vi "Graficar.vi"(8 "error in":errorcluster, 10 "group name":string, 11 "channel name":string) -> (0 "error out":errorcluster, 2 "XY Graph":cluster{timestamp[], dbl[]}(graph), 3 "semaphore out":T1)   [LabVIEW 2015]
panel:
  out "x-y":i32
  out "count":i32
  out "Boolean":bool
  out "offset":i32
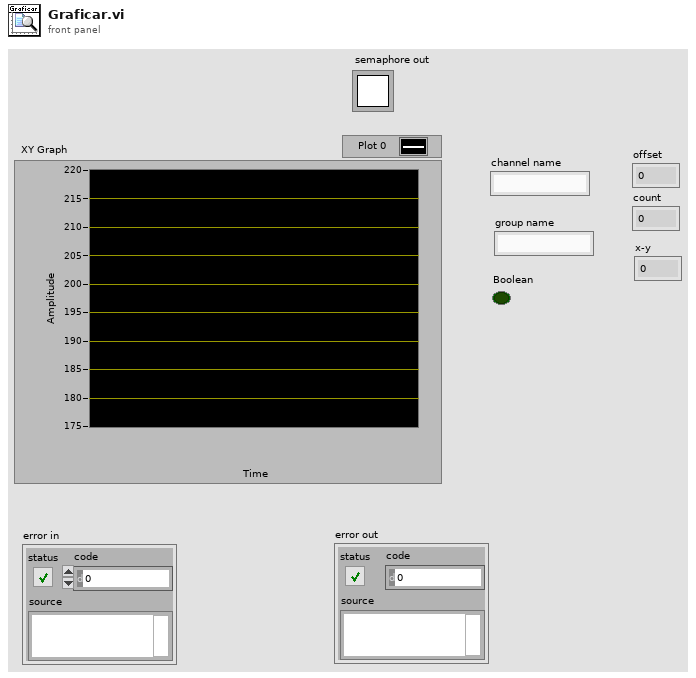
[diagram p1: front panel]
types:
  T1 = typedef "Semaphore RefNum" = refnum<k1>
  T2 = cluster{"tdms control out":refnum<k34>, "tdms historial out":refnum<k34>, "tdms sinc out":refnum<k34>}
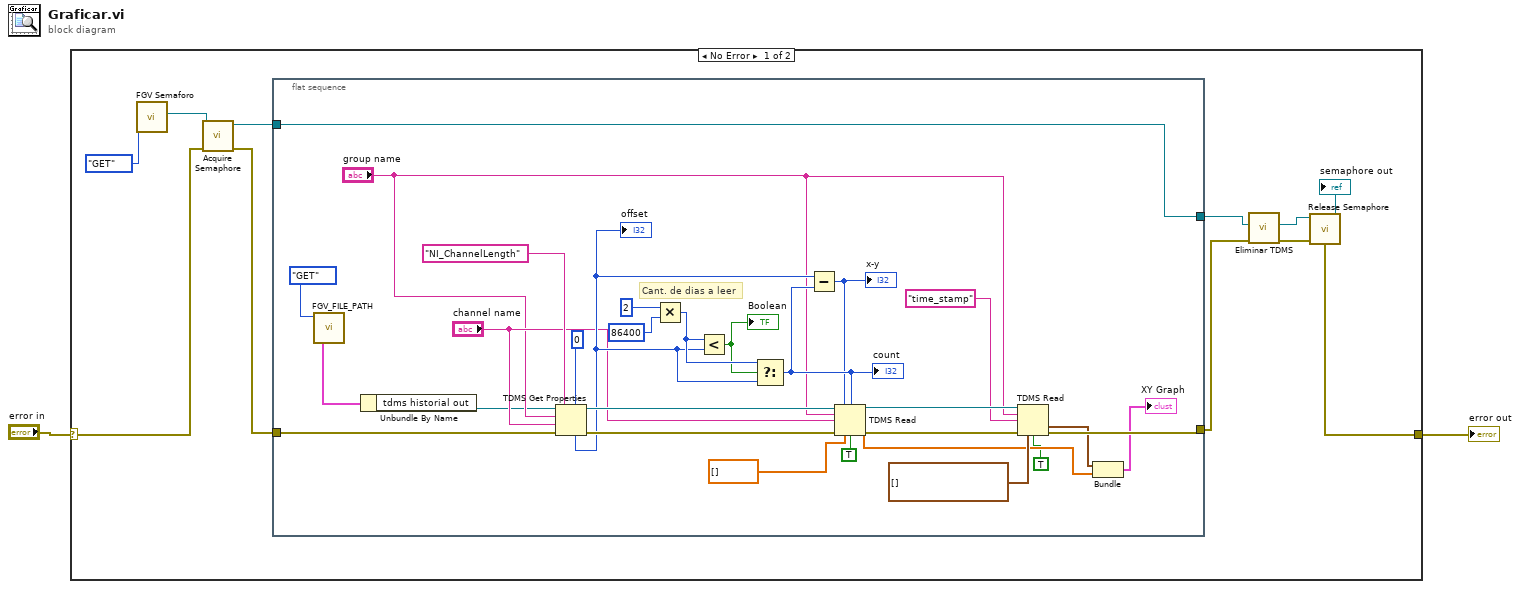
[diagram p0: block diagram]
diagram:
  n1 = case shown="No Error" "error in" {
    selector: "error in" -> [w10 w43]
    tunnel: [w9 w43] -> w1
    frame No Error {
      n2 = call "FGV Semaforo.vi"("Function"=enum16{"GET", "SET"}."GET") -> ("semaphore out"=w11:T1)  [unwired: 10 in]
      n3 = call <vilib>:"Acquire Semaphore.vi"("error in (no error)"=w10, "semaphore"=w11) -> ("error out"=w8:errorcluster, "semaphore out"=w7:T1)  [unwired: 3 in, 1 out]
      n4 = flat-sequence {
        tunnel: [w42] -> w6
        tunnel: w8 -> [w15]
        tunnel: [w14] -> w5
        tunnel: w7 -> [w14]
        frame #0 {
          # "Cant. de dias a leer"
          n5 = call "FGV_FILE_PATH.vi"("Function"=enum16{"GET", "SET"}."GET") -> ("Data Out"=w17:T2)  [unwired: 10 in]
          n6 = Unbundle By Name(w17) -> ("tdms historial out"=w16:refnum<k34>)
          n7 = TDMS Get Properties(5:0, 7:"NI_ChannelLength" ("property name"), 8:w15, 9:"channel name", 10:"group name", 11:w16) -> (0:w38:errorcluster, 3:w39:refnum<k34>, 4:w34:i32)  [unwired: 3 out]
          "offset" <- w34
          n8 = Multiply(x=2, y=86400) -> (x*y=w36:i32)
          n9 = Less?(x=w36, y=w34) -> (x < y?=w35:bool)
          "Boolean" <- w35
          n10 = Select(t=w36, s=w35, f=w34) -> (s? t:f=w33:i32)
          "count" <- w33
          n11 = Subtract(x=w34, y=w33) -> (x-y=w19:i32)
          "x-y" <- w19
          n12 = TDMS Read(0:w39, 1:w19, 2:w33, 5:"group name", 7:"channel name", 11:w38, 12:dbl[] [], 13:TRUE ("return channels in file order? (F)")) -> (4:w30:refnum<k34>, 10:w25:dbl[], 15:w29:errorcluster)  [unwired: 3 out]
          n13 = TDMS Read(0:w30, 5:"group name", 7:"time_stamp" ("channel name(s) in"), 11:w29, 12:timestamp[] [], 13:TRUE ("return channels in file order? (F)")) -> (10:w26:timestamp[], 15:w42:errorcluster)  [unwired: 2 in, 4 out]
          n14 = Bundle(w26, w25) -> (→"XY Graph":cluster{timestamp[], dbl[]})  [unwired: 1 in]
        }
      }
      n15 = call "Eliminar TDMS.vi"("error in"=w6, "semaphore"=w5) -> ("error out"=w3:errorcluster, "semaphore out"=w4:T1)  [unwired: 8 in]
      n16 = call <vilib>:"Release Semaphore.vi"("error in (no error)"=w3, "semaphore"=w4) -> ("error out"=w9:errorcluster, "semaphore out"=→"semaphore out":T1)  [unwired: 4 in]
    }
    frame Error {
    }
  }
  "error out" <- w1
